vi "Load SS Outputs.vi"(8 "Ball Gatherer State":T1=enum."Positional", 10 "Load Actuator Values":T2) -> (0 "error out":errorcluster)   [LabVIEW 2015]
uses:
  Load Actuator Values.ctl
  Ball Gatherer State.ctl
  Global Variables/refnum names.vi
  Global Variables/Temp Variables.vi
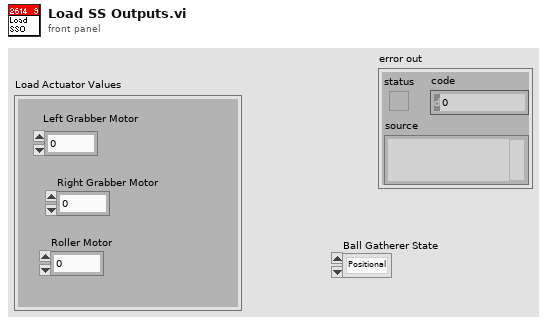
[diagram p1: front panel]
types:
  T1 = typedef "Ball Gatherer State.ctl" = enum16{"Manual", "Positional"}
  T2 = typedef "Load Actuator Values.ctl" = cluster{"Left Grabber Motor":dbl, "Right Grabber Motor":dbl, "Roller Motor":dbl}
  T3 = typedef "WPI_MotorControlDeviceRef.ctl" = cluster{"DeviceStatus":errorcluster, "Type":T4, "PWM":cluster{"PWM Channel":T5, "DeadBand":T6}, "CAN":cluster{"Device Number":u8, "Control Mode":T7, "Semaphore":T8, "Max Vout":dbl, "TalonSRX Control Mode":T9}, "Invert":bool}
  T4 = typedef "WPI_MotorControlType.ctl" = enum16{"PWM", "CAN", "CANTalonSRX"}
  T5 = typedef "FPGA_DIOPWMChannel.ctl" = enum8{"PWM 0", "PWM 1", "PWM 2", "PWM 3", "PWM 4", "PWM 5", "PWM 6", "PWM 7", "PWM 8", "PWM 9", "PWM MXP 0", "PWM MXP 1", "PWM MXP 2", "PWM MXP 3", "PWM MXP 4", "PWM MXP 5", "PWM MXP 6", "PWM MXP 7", "PWM MXP 8", "PWM MXP 9", "Invalid"}
  T6 = typedef "WPI_PWMDeadband.ctl" = cluster{"Name":string, "maxPositivePwm":i32, "minPositivePwm":i32, "centerPwm":i32, "maxNegativePwm":i32, "minNegativePwm":i32, "angularRange":u16}
  T7 = typedef "WPI_CANJaguar_ControlMode.ctl" = enum8{"Percent VBus", "Current", "Speed", "Position", "Voltage"}
  T8 = typedef "Semaphore RefNum" = refnum<k1>
  T9 = typedef "WPI_CANTalonSRX_APIControlMode.ctl" = enum8{"Percent VBus", "Speed", "Position", "Slave", "Unchanged / Invalid", "Voltage Compensation", "Current", "Motion Profile"}
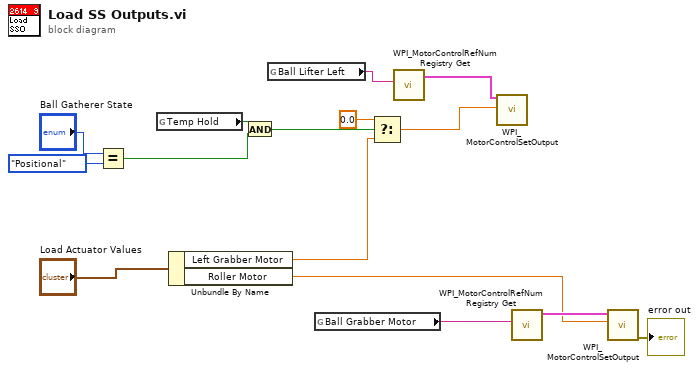
[diagram p0: block diagram]
diagram:
  n1 = Equal?(x="Ball Gatherer State", y=Ball_Gatherer_State."Positional") -> (x = y?=w8:bool)
  n2 = global read "Temp Variables.vi" "Temp Hold"() -> (w11:bool)
  n3 = Unbundle By Name("Load Actuator Values") -> ("Left Grabber Motor"=w5:dbl, "Roller Motor"=w12:dbl)
  n4 = And(x=w11, y=w8) -> (x .and. y?=w6:bool)
  n5 = global read "refnum names.vi" "Ball Lifter Left"() -> (w2:string)
  n6 = global read "refnum names.vi" "Ball Grabber Motor"() -> (w13:string)
  n7 = Select(t=0.0, s=w6, f=w5) -> (s? t:f=w1:dbl)
  n8 = call <vilib>:"WPI_MotorControlRefNum Registry Get.vi"("refnum name"=w2) -> ("MotorControlDevRef"=w3:T3)  [unwired: 9 in, 1 out]
  n9 = call <vilib>:"WPI_MotorControlSetOutput.vi"("Output"=w1, "MotorControlDevRef"=w3) -> ()  [unwired: 7 in, 3 out]
  n10 = call <vilib>:"WPI_MotorControlRefNum Registry Get.vi"("refnum name"=w13) -> ("MotorControlDevRef"=w14:T3)  [unwired: 9 in, 1 out]
  n11 = call <vilib>:"WPI_MotorControlSetOutput.vi"("Output"=w12, "MotorControlDevRef"=w14) -> ("error out"=→"error out":errorcluster)  [unwired: 7 in, 2 out]
